vi "DSF.Shared.Configuration.Framework.From JSON.vi"(8 "error in (no error)":errorcluster, 11 "Framework Configuration in":refnum<class "DSF.Shared.Configuration.Framework.lvclass">) -> (0 "error out":errorcluster, 3 "Framework Configuration out":refnum<class "DSF.Shared.Configuration.Framework.lvclass">)   [LabVIEW 2017, in "DSF.Shared.lvlib" / "DSF.Shared.Configuration.Framework.lvclass"]
uses:
  DSF.Shared.Configuration.Framework.lvclass
  Typedefs/DSF.Shared.Refactor.Typedefs.Framework Configuration.Aggregate.JSON.ctl
  Typedefs/DSF.Shared.Refactor.Typedefs.Plugin Configuration.Aggregate.JSON.ctl
  Typedefs/DSF.Shared.Typedefs.Cycle Timing Factors.ctl
  Typedefs/DSF.Shared.Refactor.Typedefs.Transfer Group Configuration.Aggregate.JSON.ctl
  Typedefs/DSF.Shared.Refactor.Typedefs.JSON.Transfer Configuration.ctl
  Typedefs/DSF.Shared.Refactor.Typedefs.JSON.Channel Array Configuration.ctl
  DSF.Shared.Configuration.Framework.lvclass/DSF.Shared.Configuration.Framework.ctl
  DSF.Shared.lvlib
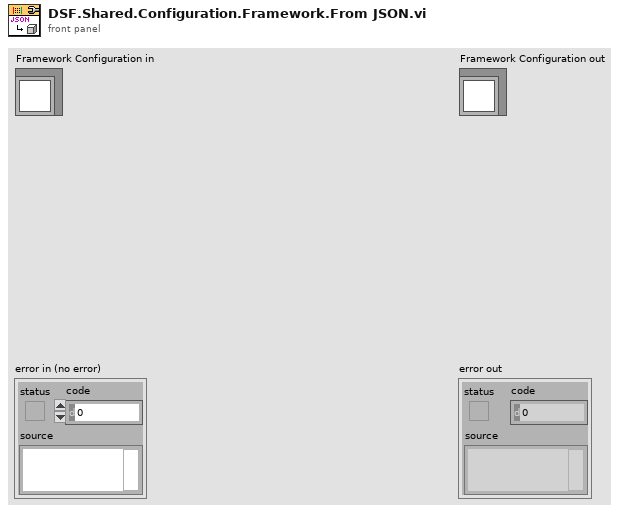
[diagram p1: front panel]
types:
  T1 = typedef "DSF.Shared.lvlib/DSF.Shared.Refactor.Typedefs.Framework Configuration.Aggregate.JSON.ctl" = cluster{"Plugins":T2[]}
  T2 = typedef "DSF.Shared.lvlib/DSF.Shared.Refactor.Typedefs.Plugin Configuration.Aggregate.JSON.ctl" = cluster{"name":string, "class":string, "cycle timing":T3, "Transfer Groups":T4[]}
  T3 = typedef "DSF.Shared.lvlib/DSF.Shared.Typedefs.Cycle Timing Factors.ctl" = cluster{"Priority":u64, "Decimation":u64, "Offset":u64}
  T4 = typedef "DSF.Shared.lvlib/DSF.Shared.Refactor.Typedefs.Transfer Group Configuration.Aggregate.JSON.ctl" = cluster{"name":string, "direction":u8, "cycle timing":T3, "Transfers":T5[]}
  T5 = typedef "DSF.Shared.lvlib/DSF.Shared.Refactor.Typedefs.JSON.Transfer Configuration.ctl" = cluster{"name":string, "byte order":u8, "channel configurations":T6[]}
  T6 = typedef "DSF.Shared.lvlib/DSF.Shared.Refactor.Typedefs.JSON.Channel Array Configuration.ctl" = cluster{"name":string, "data type":u8, "count":u64, "buffer offset":u64, "VS channel ref":u64}
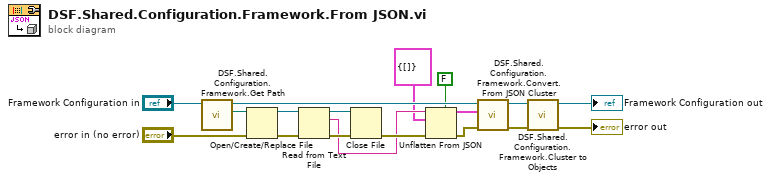
[diagram p0: block diagram]
diagram:
  n1 = call "DSF.Shared.Configuration.Framework.Get Path.vi"("Framework Configuration in"="Framework Configuration in") -> ("configuration path"=w18:path, "Framework Configuration out"=w9:refnum<class "DSF.Shared.Configuration.Framework.lvclass">)  [unwired: 9 in]
  n2 = Open/Create/Replace File(file path (use dialog)=w18, error in="error in (no error)") -> (refnum out=w16:refnum<file>, error out=w17:errorcluster)  [unwired: 4 in, 1 out]
  n3 = Read from Text File(file (use dialog)=w16, error in=w17) -> (refnum out=w15:refnum<file>, text=w10:string, error out=w14:errorcluster)  [unwired: 2 in, 1 out]
  n4 = Close File(refnum=w15, error in=w14) -> (error out=w11:errorcluster)  [unwired: 1 out]
  n5 = Unflatten From JSON(enable LabVIEW extensions? (T)=FALSE, JSON string=w10, type and defaults=T1 {"Plugins"=[]} ("Framework Config (JSON)"), error in (no error)=w11) -> (value=w6:T1, error out=w8:errorcluster)  [unwired: 3 in]
  n6 = call "DSF.Shared.Configuration.Framework.Convert.From JSON Cluster.vi"("error in (no error)"=w8, "Framework Config (JSON)"=w6, "Framework Configuration in"=w9) -> ("error out"=w4:errorcluster, "Framework Configuration out"=w5:refnum<class "DSF.Shared.Configuration.Framework.lvclass">)  [unwired: 7 in]
  n7 = call "DSF.Shared.Configuration.Framework.Cluster to Objects.vi"("error in (no error)"=w4, "Framework Configuration in"=w5) -> ("error out"=→"error out":errorcluster, "Framework Configuration out"=→"Framework Configuration out":refnum<class "DSF.Shared.Configuration.Framework.lvclass">)  [unwired: 8 in]
